vi "IO Node to IQ Data - S16.1 - 1 spc.vi"(0 "I data in":fxp<+/-,16,1>, 5 "Q data in":fxp<+/-,16,1>, 7 "I overrange":bool, 9 "Q overrange":bool) -> (4 "data":T1)   [LabVIEW 2025, in "niUSRP Rx Core v1 FPGA.lvclass"]
doc: "this VI converts ADC data to IQ data and reports ADC overrange via software register as well as inserts ADC overrange into the DSP path (aligned with the data). the first element, data[0], is the oldest sample in the array.\n\n<B>I data in:</B> specifies the real part of the data.\n\n<B>Q data in:</B> specifies the imaginary part of the data.\n\n<B>data:</B> returns a cluster of real and imaginary data.\n\n<B>I overrange:</B> indicates whether the I ADC data has overflowed.\n\n<B>Q overrange:</B> indicates whether the Q ADC data has overflowed."
uses:
  niUSRP Rx Core v1 FPGA.lvclass
  niUSRP Rx Core v1 FPGA.lvclass/niUSRP Rx Core v1 FPGA.ctl
  <instrlib>/_niInstr/DSP/v1/Shared/Public/IQ Data.ctl
  <instrlib>/_niInstr/DSP/v1/Shared/niInstr DSP v1 Shared.lvlib
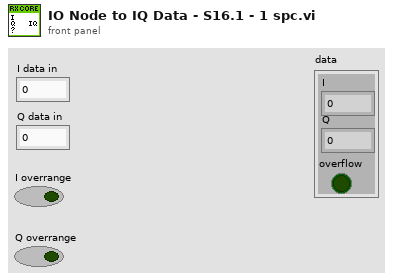
[diagram p1: front panel]
types:
  T1 = typedef "niInstr DSP v1 Shared.lvlib/IQ Data.ctl" = cluster{"I":fxp<+/-,18,1>, "Q":fxp<+/-,18,1>, "overflow":bool}
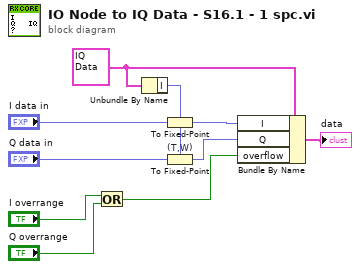
[diagram p0: block diagram]
diagram:
  w4 = T1 {"I"=0.0, "Q"=0.0, "overflow"=FALSE} ("IQ Data")
  n1 = Or(x="I overrange", y="Q overrange") -> (x .or. y?=w3:bool)
  n2 = Unbundle By Name(w4) -> ("I"=w7:fxp<+/-,18,1>)
  n3 = To Fixed-Point ("(T,W)")(fixed-point type=w7, number="I data in") -> (fixed-point=w9:fxp<+/-,18,1>)
  n4 = To Fixed-Point "(T,W)"(fixed-point type=w7, number="Q data in") -> (fixed-point=w8:fxp<+/-,18,1>)
  n5 = Bundle By Name(cluster=w4, "I"=w9, "Q"=w8, "overflow"=w3) -> (→"data":T1)
